vi "Tx Channel Page.vi"(8 "error in (no error)":errorcluster, 11 "Node Ptr":T2 format="%.0x") -> (0 "error out":errorcluster)   [LabVIEW 2019, in "UDP-Custom-Device System Explorer.lvlib"]
uses:
  UDP-Custom-Device System Explorer.lvlib
  Shared/Types/Shared - Channel Data Type.ctl
  <vilib>/NI VeriStand/Custom Device API/Custom Device Item Ref.ctl
  <vilib>/NI VeriStand/Custom Device API/Custom Device API.lvlib
  Property Accessors/Rx Channel Accessors.lvlib
  Property Accessors/Rx Channel Section Accessors.lvlib
  Shared/UDP-Custom-Device Shared.lvlib
panel:
  out "Field Index":i32
  in  "Data Type":T1
  in  "SHDocVw.IWebBrowser":refnum<k7>(container)
  in  "General Header":cluster{"Section Name":string}={"Section Name"="Tx Channel Settings"}
  in  "Description":string
  in  "Name":string
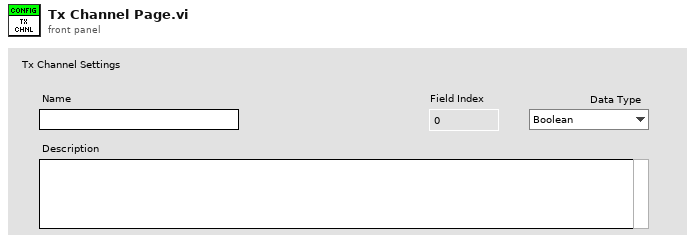
[diagram p1: front panel]
types:
  T1 = typedef "UDP-Custom-Device Shared.lvlib/Shared - Channel Data Type.ctl" = enum16{"Boolean", "Single", "Double", "I8", "I16", "I32", "I64", "U8", "U16", "U32", "U64"}
  T2 = typedef "Custom Device API.lvlib/Custom Device Item Ref.ctl" = u64
  T3 = typedef "Custom Device API.lvlib/Custom Device Item Info.ctl" = cluster{"Name":string, "Is Channel":bool, "GUID":string, "Is Waveform":bool}
  T4 = typedef "Custom Device API.lvlib/Custom Device Commands.ctl" = enum16{"Default", "Item renamed", "Shutdown", "Dynamic button pressed"}
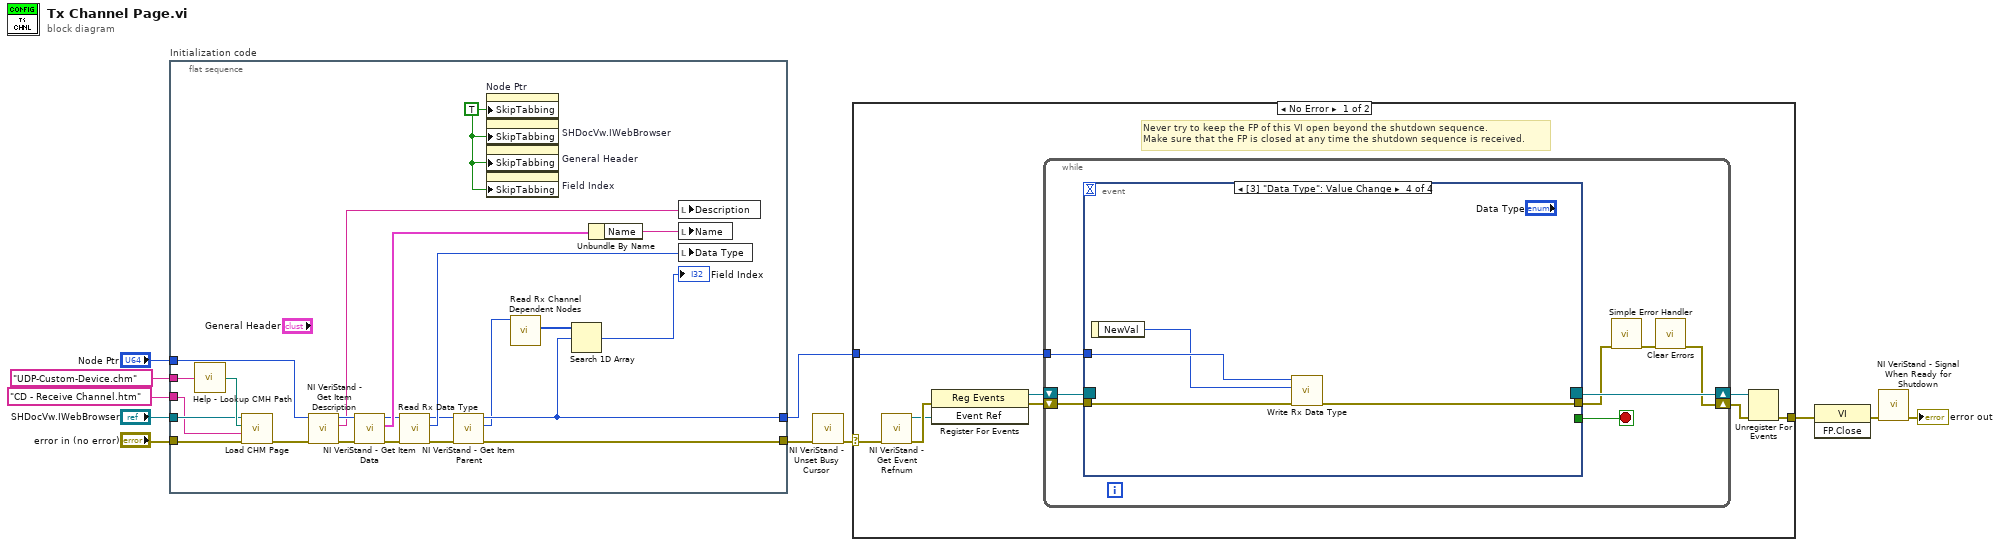
[diagram p0: block diagram]
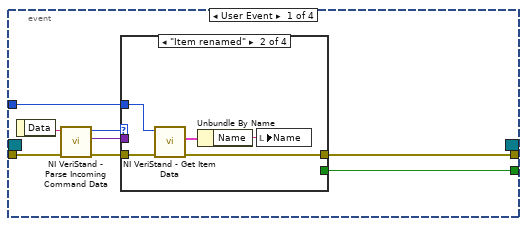
[diagram p2: hidden frame]
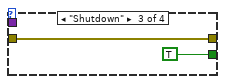
[diagram p4: hidden frame]
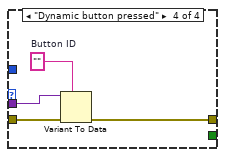
[diagram p5: hidden frame]
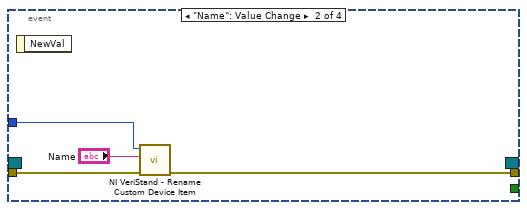
[diagram p6: hidden frame]
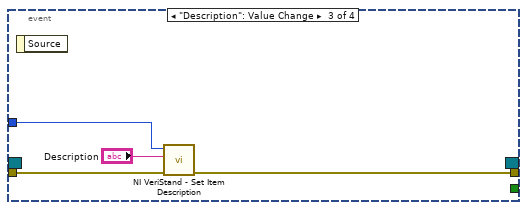
[diagram p7: hidden frame]
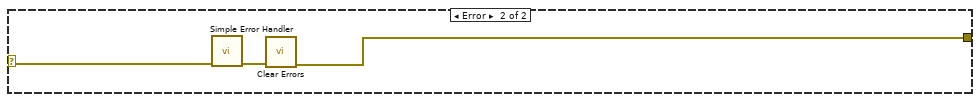
[diagram p8: hidden frame]
diagram:
  n1 = flat-sequence "Initialization code" {
    tunnel: "error in (no error)" -> [w27]
    tunnel: "Node Ptr" -> [w31]
    tunnel: [w18] -> w7
    tunnel: [w16] -> w4
    tunnel: "SHDocVw.IWebBrowser" -> [w25]
    tunnel: "CD - Receive Channel.htm" ("CD_CHM_Section") -> [w24]
    tunnel: "UDP-Custom-Device.chm" ("CD_CHM_FileName") -> [w26]
    frame #0 {
      w14 = TRUE ("Skip When Tabbing")
      n2 = call "Help - Lookup CMH Path.vi"("Main CMH File"=w26) -> ("Compiled CMH Path"=w28:path)
      n3 = call <vilib>:"Load CHM Page.vi"("error in (no error)"=w27, "HTML File"=w24, "Compiled CHM Path"=w28, "Web Browser Reference"=w25) -> ("error out"=w23:errorcluster)  [unwired: 7 in]
      n4 = call <vilib>:"NI VeriStand - Get Item Description.vi"("error in (no error)"=w23, "Item Ref in"=w31) -> ("error out"=w33:errorcluster, "Description"=w29:string, "Item Ref out"=w34:T2)  [unwired: 7 out]
      n5 = call <vilib>:"NI VeriStand - Get Item Data.vi"("error in (no error)"=w33, "Item Ref in"=w34) -> ("error out"=w21:errorcluster, "Item Info"=w32:T3, "Item Ref out"=w22:T2)  [unwired: 7 out]
      n6 = call "Read Rx Data Type.vi"("error in (no error)"=w21, "Node Ptr"=w22) -> ("error out"=w19:errorcluster, "Data Type"=w20:T1, "Node Ptr out"=w17:T2)  [unwired: 7 in]
      n7 = call <vilib>:"NI VeriStand - Get Item Parent.vi"("error in (no error)"=w19, "Item Ref in"=w17) -> ("error out"=w18:errorcluster, "Parent Ref"=w13:T2, "Item Ref out"=w16:T2)  [unwired: 6 in, 1 out]
      n8 = property on="Node Ptr" class="DigNum (strict)"("SkipTabbing"=w14) -> ()  [unwired: 2 in, 2 out]
      n9 = property on="SHDocVw.IWebBrowser" class="AXCont"("SkipTabbing"=w14) -> ()  [unwired: 2 in, 2 out]
      n10 = property on="General Header" class="Clust (strict)"("SkipTabbing"=w14) -> ()  [unwired: 2 in, 2 out]
      n11 = property on="Field Index" class="DigNum (strict)"("SkipTabbing"=w14) -> ()  [unwired: 2 in, 2 out]
      n12 = call "Read Rx Channel Dependent Nodes.vi"("Node Ptr"=w13) -> ("Dependent Node Refs"=w12:T2[])  [unwired: 8 in, 2 out]
      n13 = Search 1D Array(1D array=w12, element=w16) -> (index of element=→"Field Index":i32)  [unwired: 1 in]
      n14 = Unbundle By Name(w32) -> ("Name"=w30:string)
      n15 = local write "Description"(w29) -> ()
      n16 = local write "Name"(w30) -> ()
      n17 = local write "Data Type"(w20) -> ()
    }
  }
  n18 = call <vilib>:"NI VeriStand - Unset Busy Cursor.vi"("error in (no error)"=w7) -> ("error out"=w6:errorcluster)  [unwired: 10 out]
  n19 = case shown="No Error" w6 {
    selector: w6 -> [w35 w86]
    tunnel: [w40 w84] -> w11
    tunnel: w4 -> [w36 _]
    frame No Error {
      # "Never try to keep the FP of this VI open beyond the shutdown sequence.\nMake sure that the FP is closed at any time the shutdown sequence is received."
      n20 = call <vilib>:"NI VeriStand - Get Event Refnum.vi"("error in (no error)"=w35) -> ("error out"=w43:errorcluster, "Event Ref"=w39:refnum<user-event>)  [unwired: 9 out]
      n21 = register-events(error in=w43, w39) -> (reference out=w37:refnum<event-registration>, error out=w38:errorcluster)  [unwired: 1 in]
      n22 = while {
        tunnel: w36 -> [w47]
        shift-right: [w44] -> w41
        shift-left: w38 -> [w50]
        shift-right: [w51] -> w42
        shift-left: w37 -> [w49]
        stop <- w48 stop-if-true
        n23 = event shown="[3] \"Data Type\": Value Change" {
          selector: w49 -> [_ _ _ _]
          dyn-events: [_ _ _ _] -> w51
          timeout: _ -> [_ _ _ _]
          tunnel: w50 -> [w59 w75 w78 w81]
          tunnel: [w55 _ _ _] -> w48
          tunnel: [w54 w74 w77 w80] -> w46
          tunnel: w47 -> [w53 w73 w79 w83]
          event User Event {
            n24 = event-data() -> ("Data"=w58:string)  [unwired: 1 out]
            n25 = call <vilib>:"NI VeriStand - Parse Incoming Command Data.vi"("error in (no error)"=w59, "Incoming data"=w58) -> ("error out"=w57:errorcluster, "Outgoing data"=w52:variant, "Action"=w56:T4)  [unwired: 7 out]
            n26 = case shown="\"Item renamed\"" w56 {
              tunnel: w57 -> [w60 w65 w66 w71]
              tunnel: [_ _ TRUE _] -> w55
              tunnel: [w60 w62 w66 w68] -> w54
              tunnel: w53 -> [_ w64 _ _]
              tunnel: w52 -> [_ _ _ w70]
              frame "Default", Default {
              }
              frame "Item renamed" {
                n27 = call <vilib>:"NI VeriStand - Get Item Data.vi"("error in (no error)"=w65, "Item Ref in"=w64) -> ("error out"=w62:errorcluster, "Item Info"=w63:T3)  [unwired: 8 out]
                n28 = Unbundle By Name(w63) -> ("Name"=w61:string)
                n29 = local write "Name"(w61) -> ()
              }
              frame "Shutdown" {
              }
              frame "Dynamic button pressed" {
                w69 = ""  # Button ID
                n30 = Variant To Data(error in=w71, type=w69, Variant=w70) -> (error out=w68:errorcluster)  [unwired: 1 out]
              }
            }
          }
          event "Name": Value Change {
            n31 = event-data() -> ()  [unwired: 2 out]
            n32 = call <vilib>:"NI VeriStand - Rename Custom Device Item.vi"("error in (no error)"=w75, "New Name"="Name", "Item Ref in"=w73) -> ("error out"=w74:errorcluster)  [unwired: 1 in, 7 out]
          }
          event "Description": Value Change {
            n33 = event-data() -> ()  [unwired: 2 out]
            n34 = call <vilib>:"NI VeriStand - Set Item Description.vi"("error in (no error)"=w78, "Description"="Description", "Item Ref in"=w79) -> ("error out"=w77:errorcluster)  [unwired: 8 out]
          }
          event Value Change {
            n35 = event-data() -> ("NewVal"=w82:T1)  [unwired: 1 out]
            n36 = call "Write Rx Data Type.vi"("error in (no error)"=w81, "Data Type"=w82, "Node Ptr"=w83) -> ("error out"=w80:errorcluster)  [unwired: 7 in, 1 out]
          }
        }
        n37 = call <vilib>:"Simple Error Handler.vi"("error in (no error)"=w46) -> ("error out"=w45:errorcluster)  [unwired: 1 in, 7 out]
        n38 = call <vilib>:"Clear Errors.vi"("error in (no error)"=w45) -> ("error out"=w44:errorcluster)  [unwired: 1 in, 5 out]
      }
      n39 = Unregister For Events(event registration refnum=w42, error in=w41) -> (error out=w40:errorcluster)
    }
    frame Error {
      n40 = call <vilib>:"Simple Error Handler.vi"("error in (no error)"=w86) -> ("error out"=w85:errorcluster)  [unwired: 1 in, 7 out]
      n41 = call <vilib>:"Clear Errors.vi"("error in (no error)"=w85) -> ("error out"=w84:errorcluster)  [unwired: 1 in, 5 out]
    }
  }
  n42 = invoke class="VI" method="FP.Close"(error in=w11) -> (error out=w10:errorcluster)  [unwired: 2 in, 2 out]
  n43 = call <vilib>:"NI VeriStand - Signal When Ready for Shutdown.vi"("error in (no error)"=w10) -> ("error out"=→"error out":errorcluster)  [unwired: 10 out]
